vi "Initialize Sessions - NSess.vi"(6 "initialize and close session behavior":T2, 7 "simulate (F)":bool, 8 "error in":errorcluster, 9 "reset device (T)":bool=TRUE, 10 "topology name":T1="Configured Topology", 11 "session reservation in":refnum<class "Session Reservation.lvclass">) -> (0 "error out":errorcluster, 1 "channel lists":string[](array[string]), 2 "sessions":refnum<class "Session Factory.lvclass">[](array[class]), 3 "session reservation out":refnum<class "Session Reservation.lvclass">)   [LabVIEW 2021, in "Session Management niSwitch.lvlib"]
uses:
  Session Management niSwitch.lvlib
  Session Factory/Session Factory.lvclass
  ed19bd00-a53f-4c28-bc2f-0276bdd05363.vi
  <vilib>/Plug-In SDKs/Clients/Session Management V1/Session Reservation/Session Reservation.lvclass
  <vilib>/Plug-In SDKs/Clients/Session Management V1/Session Reservation/Initialize and Close Session Behavior.ctl
  <instrlib>/niSwitch/niSwitch.llb/niSwitch Topologies.ctl
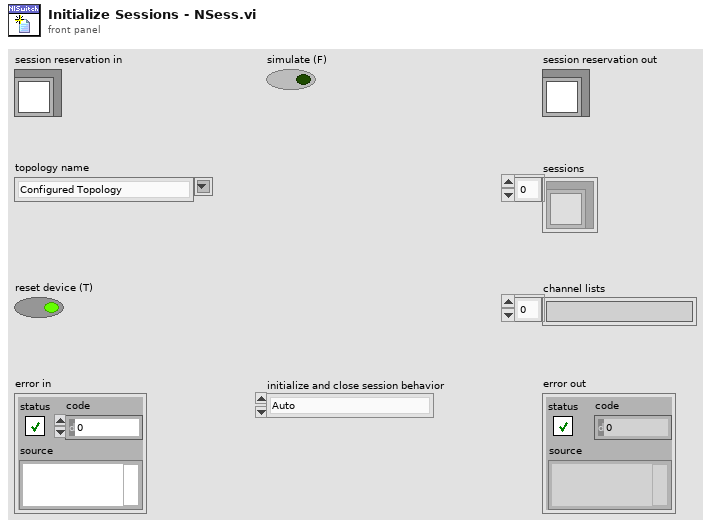
[diagram p1: front panel]
types:
  T1 = typedef "niSwitch Topologies.ctl" = string
  T2 = typedef "NI Session Management V1 Client.lvlib/Session Reservation.lvclass/Initialize and Close Session Behavior.ctl" = enum16{"Auto", "Initialize and Close", "Attach and Detach", "Initialize and Detach", "Attach and Close"}
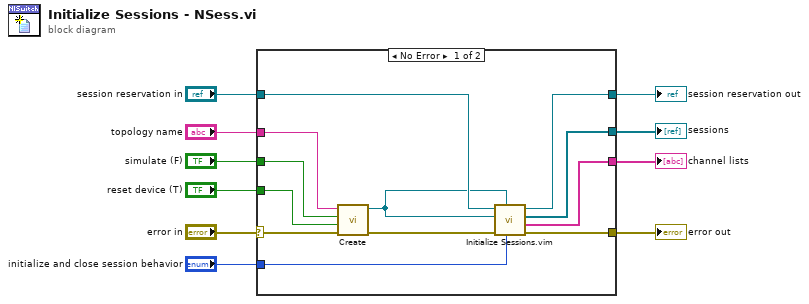
[diagram p0: block diagram]
diagram:
  n1 = case shown="No Error" "error in" {
    selector: "error in" -> [w18 w23]
    tunnel: [w20 w24] -> w10
    tunnel: "session reservation in" -> [w21 w24]
    tunnel: "initialize and close session behavior" -> [w17 _]
    tunnel: "topology name" -> [w16 _]
    tunnel: "simulate (F)" -> [w15 _]
    tunnel: "reset device (T)" -> [w14 _]
    tunnel: [w13 w23] -> w3
    tunnel: [w12 _] -> w1
    tunnel: [w11 _] -> w2
    frame No Error {
      n2 = call "Create.vi"("error in"=w18, "reset device"=w14, "simulate"=w15, "topology name"=w16) -> ("error out"=w22:errorcluster, "session factory out"=w19:refnum<class "Session Factory.lvclass">)  [unwired: 6 in]
      n3 = call "Initialize Sessions.vim"("initialize and close session behavior"=w17, "session type"=w19, "error in"=w22, "session factory"=w19, "session reservation in"=w21) -> ("error out"=w13:errorcluster, "channel lists"=w11:string[], "sessions"=w12:refnum<class "Session Factory.lvclass">[], "session reservation out"=w20:refnum<class "Session Reservation.lvclass">)  [unwired: 3 in]
    }
    frame Error {
    }
  }
  "session reservation out" <- w10
  "error out" <- w3
  "sessions" <- w1
  "channel lists" <- w2
